vi "MICSD Search for Implant.vi"(0 "VISA Resource Name":refnum<visa-resource-name>, 1 "Search Time (mS)":u32=3000, 2 "Existing MICS IDs":u32[](array[numeric]), 5 "Enable Watchdog?(T)":bool=TRUE, 7 "Any Company?(T)":bool=TRUE, 9 "Any Implant?(T)":bool=TRUE, 11 "error in (no error)":errorcluster, 12 "Mode":T1(ring)) -> (4 "dup VISA Resource Name":refnum<visa-resource-name>, 6 "Device Found?":bool, 8 "Detected MICS IDs":u32[](array[numeric]) format="%06x", 15 "error out":errorcluster)   [LabVIEW 2020]
uses:
  <vilib>/Instr/_visa.llb/VISA Configure Serial Port (Instr).vi
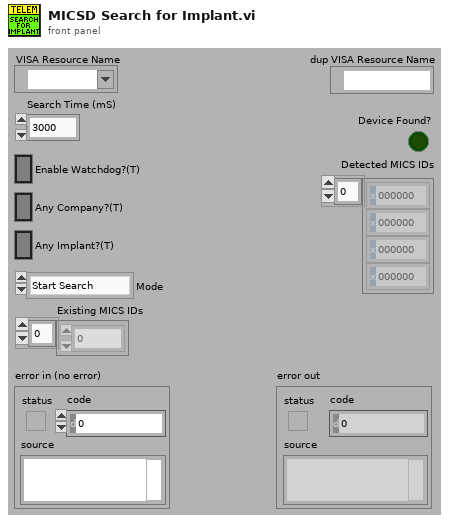
[diagram p1: front panel]
types:
  T1 = enum16{"Start Search", "Continue Search", "End Search"}
  T2 = cluster{"Command Token":u8, "Length":u16, "Pack Data":u8[]}
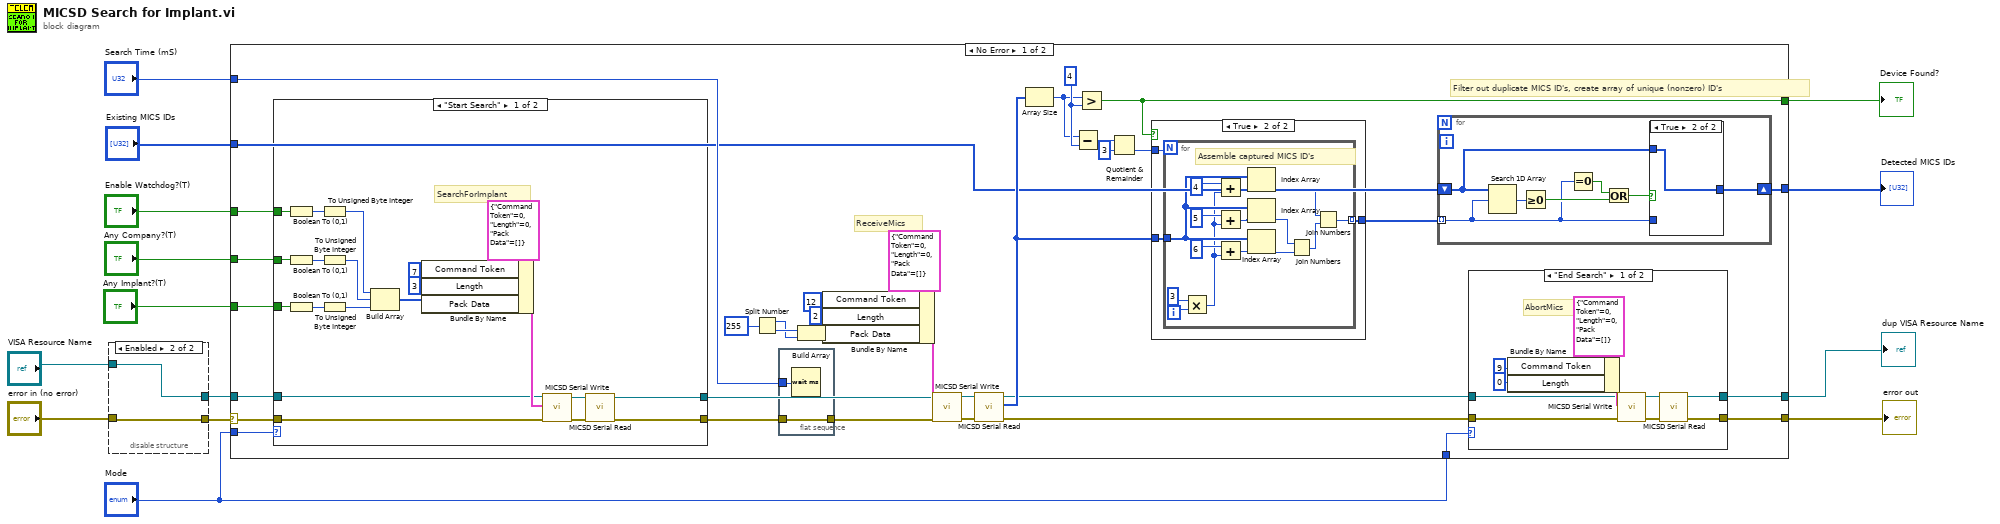
[diagram p0: block diagram]
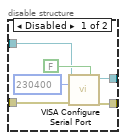
[diagram p2: hidden frame]
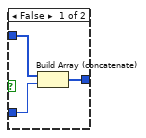
[diagram p5: hidden frame]
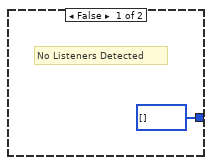
[diagram p6: hidden frame]
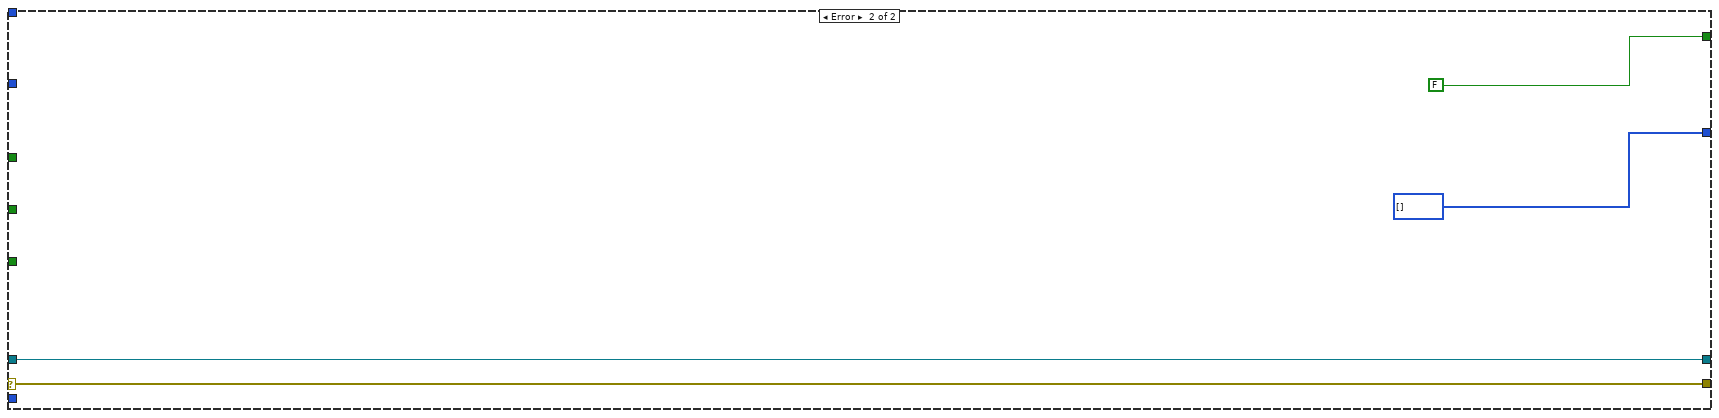
[diagram p7: hidden frame]
diagram:
  n1 = disable-structure shown="Enabled" {
    disable-tunnel: [w18 w21] -> w8
    disable-tunnel: [w17 w22] -> w7
    disable-tunnel: "VISA Resource Name" -> [w16 w22]
    disable-tunnel: "error in (no error)" -> [w15 w21]
    frame Disabled {
      n2 = call-poly "VISA Configure Serial Port"("VISA resource name"=w16, "Enable Termination\nChar (T)"=FALSE ("Enable Termination\nChar (T)"), "baud rate (9600)"=u32 230400, "error in (no error)"=w15) -> ("VISA resource name out"=w17:refnum<visa-resource-name>, "error out"=w18:errorcluster)  [unwired: 10 in]
    }
    frame Enabled {
    }
  }
  n3 = case shown="No Error" w8 {
    selector: w8 -> [w56 w124]
    tunnel: w7 -> [w57 w125]
    tunnel: "Enable Watchdog?(T)" -> [w55 _]
    tunnel: "Any Company?(T)" -> [w54 _]
    tunnel: "Any Implant?(T)" -> [w53 _]
    tunnel: "Search Time (mS)" -> [w26 _]
    tunnel: [w42 w124] -> w3
    tunnel: [w41 w125] -> w4
    tunnel: [w47 FALSE] -> w10
    tunnel: [w29 u32[] []] -> w9
    tunnel: "Mode" -> [w28 _]
    tunnel: "Mode" -> [w27 _]
    tunnel: "Existing MICS IDs" -> [w23 _]
    frame No Error {
      w33 = u16 4 ("Length")
      # "Filter out duplicate MICS ID's, create array of unique (nonzero) ID's"
      # "ReceiveMics"
      n4 = case shown="\"Start Search\"" w28 {
        tunnel: w57 -> [w75 w81]
        tunnel: w56 -> [w74 w80]
        tunnel: w55 -> [w73 _]
        tunnel: w54 -> [w72 _]
        tunnel: w53 -> [w71 _]
        tunnel: [w63 w81] -> w43
        tunnel: [w60 w80] -> w25
        frame "Start Search" {
          # "SearchForImplant"
          n5 = Boolean To (0,1)(Boolean=w73) -> (0, 1=w70:i16)
          n6 = Boolean To (0,1)(Boolean=w72) -> (0, 1=w69:i16)
          n7 = Boolean To (0,1)(Boolean=w71) -> (0, 1=w68:i16)
          n8 = To Unsigned Byte Integer(number=w70) -> (unsigned 8bit integer=w67:u8)
          n9 = To Unsigned Byte Integer(number=w69) -> (unsigned 8bit integer=w66:u8)
          n10 = To Unsigned Byte Integer(number=w68) -> (unsigned 8bit integer=w65:u8)
          n11 = Build Array(w67, w66, w65) -> (w64:u8[])
          n12 = Bundle By Name(cluster=T2 {"Command Token"=0, "Length"=0, "Pack Data"=[]} ("Write Data"), "Command Token"=u8 7, "Length"=u16 3, "Pack Data"=w64) -> (w79:T2)
          n13 = call "MICSD Serial Write.vi"("error in (no error)"=w74, "Write Data"=w79, "VISA Resource Name"=w75) -> ("error out"=w61:errorcluster, "DUP Visa Resource Name"=w62:refnum<visa-resource-name>)  [unwired: 7 in]
          n14 = call "MICSD Serial Read.vi"("error in (no error)"=w61, "VISA Resource Name"=w62) -> ("error out"=w60:errorcluster, "DUP Visa Resource Name"=w63:refnum<visa-resource-name>)  [unwired: 7 in, 1 out]
        }
        frame "Continue Search", Default {
        }
      }
      n15 = Split Number(x=u16 255 ("Command Token")) -> (hi(x)=w37:u8, lo(x)=w38:u8)
      n16 = flat-sequence {
        tunnel: w26 -> [w59]
        tunnel: w25 -> [w58]
        tunnel: [w58] -> w24
        frame #0 {
          n17 = Wait (ms)(milliseconds to wait=w59) -> ()  [unwired: 1 out]
        }
      }
      n18 = Build Array(w38, w37) -> (w48:u8[])
      n19 = Bundle By Name(cluster=T2 {"Command Token"=0, "Length"=0, "Pack Data"=[]} ("Write Data"), "Command Token"=u8 12, "Length"=u16 2, "Pack Data"=w48) -> (w52:T2)
      n20 = call "MICSD Serial Write.vi"("error in (no error)"=w24, "Write Data"=w52, "VISA Resource Name"=w43) -> ("error out"=w35:errorcluster, "DUP Visa Resource Name"=w34:refnum<visa-resource-name>)  [unwired: 7 in]
      n21 = call "MICSD Serial Read.vi"("error in (no error)"=w35, "VISA Resource Name"=w34) -> ("error out"=w40:errorcluster, "Read Data"=w44:u8[], "DUP Visa Resource Name"=w39:refnum<visa-resource-name>)  [unwired: 7 in]
      n22 = Array Size(array=w44) -> (size(s)=w32:i32)
      n23 = Subtract(x=w32, y=w33) -> (x-y=w31:i32)
      n24 = Greater?(x=w32, y=w33) -> (0:w47:bool)
      n25 = Quotient & Remainder(x=w31, y=u16 3 ("Length")) -> (floor(x/y)=w46:i32)  [unwired: 1 out]
      n26 = case shown="True" w47 {
        tunnel: w46 -> [_ w108]
        tunnel: w44 -> [_ w107]
        tunnel: [u32[] [] w106] -> w30
        frame False {
          # "No Listeners Detected"
        }
        frame True {
          n27 = for {
            N: w108 -> [_]
            tunnel: w107 -> [w121]
            tunnel: [w116] -> w106 mode=indexing
            i -> [w123]
            # "Assemble captured MICS ID's"
            n28 = Multiply(x=u16 3 ("Length"), y=w123) -> (x*y=w112:i32)
            n29 = Add(x=u16 4 ("Length"), y=w112) -> (x+y=w111:i32)
            n30 = Add(x=u16 5 ("Length"), y=w112) -> (x+y=w110:i32)
            n31 = Add(x=u16 6 ("Length"), y=w112) -> (x+y=w109:i32)
            n32 = Index Array(array=w121, index=w111) -> (element=w117:u8)
            n33 = Index Array(array=w121, index=w110) -> (element=w119:u8)
            n34 = Index Array(array=w121, index=w109) -> (element=w120:u8)
            n35 = Join Numbers(hi=w119, lo=w120) -> ((hi.lo)=w118:u16)
            n36 = Join Numbers(hi=w117, lo=w118) -> ((hi.lo)=w116:u32)
          }
        }
      }
      n37 = for {
        tunnel: w30 -> [w94] mode=indexing
        shift-right: [w100] -> w29
        shift-left: w23 -> [w96]
        n38 = Search 1D Array(1D array=w96, element=w94) -> (index of element=w97:i32)  [unwired: 1 in]
        n39 = Greater Or Equal To 0?(x=w97) -> (x >= 0?=w95:bool)
        n40 = Equal To 0?(x=w94) -> (x = 0?=w98:bool)
        n41 = Or(x=w98, y=w95) -> (x .or. y?=w99:bool)
        n42 = case shown="True" w99 {
          tunnel: w94 -> [w103 _]
          tunnel: [w102 w104] -> w100
          tunnel: w96 -> [w101 w104]
          frame False {
            n43 = Build Array (concatenate)(w101, w103) -> (w102:u32[])
          }
          frame True {
          }
        }
      }
      n44 = case shown="\"End Search\"" w27 {
        tunnel: [w88 w92] -> w42
        tunnel: [w87 w93] -> w41
        tunnel: w40 -> [w86 w92]
        tunnel: w39 -> [w84 w93]
        frame "End Search" {
          # "AbortMics"
          n45 = Bundle By Name(cluster=T2 {"Command Token"=0, "Length"=0, "Pack Data"=[]} ("Write Data"), "Command Token"=u8 9, "Length"=u16 0) -> (w91:T2)
          n46 = call "MICSD Serial Write.vi"("error in (no error)"=w86, "Write Data"=w91, "VISA Resource Name"=w84) -> ("error out"=w82:errorcluster, "DUP Visa Resource Name"=w83:refnum<visa-resource-name>)  [unwired: 7 in]
          n47 = call "MICSD Serial Read.vi"("error in (no error)"=w82, "VISA Resource Name"=w83) -> ("error out"=w88:errorcluster, "DUP Visa Resource Name"=w87:refnum<visa-resource-name>)  [unwired: 7 in, 1 out]
        }
        frame "Continue Search", Default {
        }
      }
    }
    frame Error {
    }
  }
  "Detected MICS IDs" <- w9
  "dup VISA Resource Name" <- w4
  "error out" <- w3
  "Device Found?" <- w10
